vi "GetIndicatorPath.vi"(11 "Error indicator type":T1) -> (2 "Exists?":bool, 3 "Path":path)   [LabVIEW 2017, in "ErrorStructureDrawer.lvlib"]
doc: "Returns the path to the error indicator for the specified type.\n\nIf an unhandled type is selected (e.g. System), or if no indicator is found for the specified type, then the path to the Modern error indicator is returned."
uses:
  ErrorStructureDrawer.lvlib
  Controls/ErrorControlType.ctl
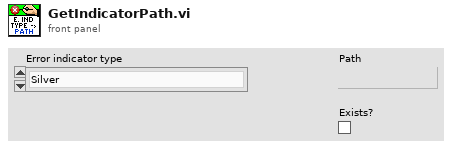
[diagram p1: front panel]
types:
  T1 = typedef "ErrorStructureDrawer.lvlib/ErrorControlType.ctl" = enum16{"Silver", "Modern", "Classic", "LabVIEW default", "NXG"}
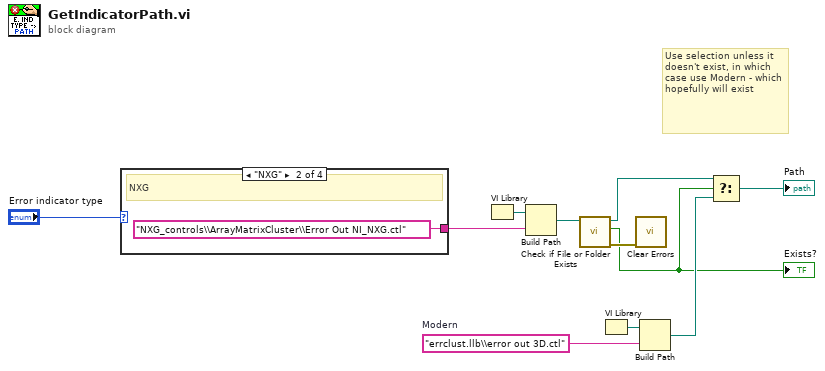
[diagram p0: block diagram]
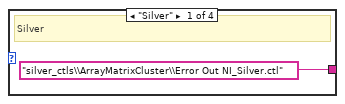
[diagram p2: hidden frame]
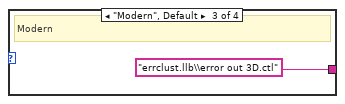
[diagram p3: hidden frame]
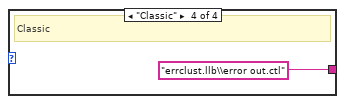
[diagram p4: hidden frame]
diagram:
  w7 = "errclust.llb\\error out 3D.ctl"  # Modern
  # "Use selection unless it doesn't exist, in which case use Modern - which hopefully will exist"
  n1 = case shown="\"NXG\"" "Error indicator type" {
    tunnel: ["silver_ctls\\ArrayMatrixCluster\\Error Out NI_Silver.ctl" ("name or relative path") "NXG_controls\\ArrayMatrixCluster\\Error Out NI_NXG.ctl" ("name or relative path") "errclust.llb\\error out 3D.ctl" ("name or relative path") "errclust.llb\\error out.ctl" ("name or relative path")] -> w1
    frame "Silver" {
      # "Silver"
    }
    frame "NXG" {
      # "NXG"
    }
    frame "Modern", Default {
      # "Modern"
    }
    frame "Classic" {
      # "Classic"
    }
  }
  n2 = VI Library() -> (path=w9:path)
  n3 = Build Path(base path=w9, name or relative path=w1) -> (appended path=w10:path)
  n4 = call <vilib>:"Check if File or Folder Exists.vi"("path"=w10) -> ("error out"=w11:errorcluster, "file or folder exists?"=w3:bool, "dup path"=w4:path)  [unwired: 8 in]
  "Exists?" <- w3
  n5 = VI Library() -> (path=w8:path)
  n6 = call <vilib>:"Clear Errors.vi"("error in (no error)"=w11) -> ()  [unwired: 5 in, 2 out]
  n7 = Build Path(base path=w8, name or relative path=w7) -> (appended path=w6:path)
  n8 = Select(t=w4, s=w3, f=w6) -> (s? t:f=→"Path":path)
